vi "WPI_CANJaguar_SetMotor.vi"(8 "error in (no error)":errorcluster, 9 "options":u8, 10 "Output":dbl, 11 "MotorControlDevRef":T1={"DeviceStatus"={"status"=FALSE, "code"=0, "source"=""}, "Type"=enum."PWM", "PWM"={"PWM Channel"=enum."Invalid", "DeadBand"={"Name"="", "maxPositivePwm"=0, "minPositivePwm"=0, "centerPwm"=0, "maxNegativePwm"=0, "minNegativePwm"=0, "angularRange"=0}}, "CAN"={"Device Number"=0, "SetOutput VI Ref"=variant(refnum<vi> refnum), "GetOutput VI Ref"=variant(refnum<vi> refnum), "Enable VI Ref"=variant(refnum<vi> refnum), "Disable VI Ref"=variant(refnum<vi> refnum), "Data"=variant}, "Invert"=FALSE}) -> (0 "error out":errorcluster, 2 "Motor Output":dbl, 3 "MotorControlDevRef":T1={"DeviceStatus"={"status"=FALSE, "code"=0, "source"=""}, "Type"=enum."PWM", "PWM"={"PWM Channel"=enum."Invalid", "DeadBand"={"Name"="", "maxPositivePwm"=0, "minPositivePwm"=0, "centerPwm"=0, "maxNegativePwm"=0, "minNegativePwm"=0, "angularRange"=0}}, "CAN"={"Device Number"=0, "SetOutput VI Ref"=variant(refnum<vi> refnum), "GetOutput VI Ref"=variant(refnum<vi> refnum), "Enable VI Ref"=variant(refnum<vi> refnum), "Disable VI Ref"=variant(refnum<vi> refnum), "Data"=variant}, "Invert"=FALSE})   [LabVIEW 2016]
doc: "Specifies the output value or set-point for the motor controller.\n\nIf you use a motor controller connected to PWM, the scaled value can range from -1.0 to 1.0.\n\nIf you use a CAN Jaguar, the scale and the units depend on the mode the Jaguar is in. In <B>Percent VBus</B> mode, the range is the same as the PWM interface. In <B>Voltage</B>, <B>Current</B>, <B>Speed</B>, and <B>Position</B> modes, the <B>Output</B> is specified in engineering units (Volts, Amps, Rotations/Minute, and Rotations respectively).\n\nIf you use a CAN Talon SRX, the scale and the units depend on the mode the Talon SRXis in. In <B>Percent VBus</B> mode, the range is the same as the PWM interface. In <B>Speed</B>, and <B>Position</B> modes, the <B>Output</B> is specified in raw sensor units (ticks and ticks / 100 ms respectively).\n\nThis software is licensed. Open the labview\\readme\\WPI Robotics Library Open Source License.txt file for more information."
uses:
  <vilib>/Rock Robotics/WPI/MotorControl/WPI_MotorControlDeviceRef.ctl
  <vilib>/Rock Robotics/WPI/MotorControl/WPI_MotorControlType.ctl
  <vilib>/Rock Robotics/SystemInterfaces/DIO/FPGA_DIOPWMChannel.ctl
  <vilib>/Rock Robotics/WPI/PWM/WPI_PWMDeadband.ctl
  <vilib>/Rock Robotics/WPI/ThirdParty/CanMotor/CAN Jaguar/SubVIs/WPI_CANJaguar_RefNumData.ctl
  <vilib>/Rock Robotics/WPI/ThirdParty/CanMotor/CAN Jaguar/SubVIs/WPI_CANJaguar_ControlMode.ctl
  <vilib>/Rock Robotics/WPI/ThirdParty/CanMotor/CAN Jaguar/SubVIs/WPI_CAN_TokenMessageIDs.ctl
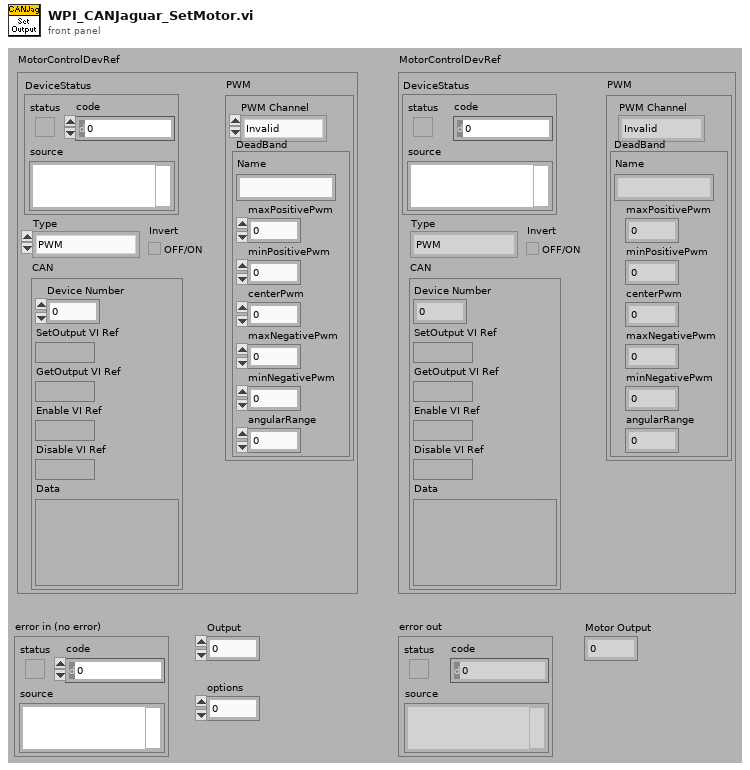
[diagram p1: front panel]
types:
  T1 = typedef "WPI_MotorControlDeviceRef.ctl" = cluster{"DeviceStatus":errorcluster, "Type":T2, "PWM":cluster{"PWM Channel":T3, "DeadBand":T4}, "CAN":cluster{"Device Number":u8, "SetOutput VI Ref":variant, "GetOutput VI Ref":variant, "Enable VI Ref":variant, "Disable VI Ref":variant, "Data":variant}, "Invert":bool}
  T2 = typedef "WPI_MotorControlType.ctl" = enum16{"PWM", "CAN"}
  T3 = typedef "FPGA_DIOPWMChannel.ctl" = enum8{"PWM 0", "PWM 1", "PWM 2", "PWM 3", "PWM 4", "PWM 5", "PWM 6", "PWM 7", "PWM 8", "PWM 9", "PWM MXP 0", "PWM MXP 1", "PWM MXP 2", "PWM MXP 3", "PWM MXP 4", "PWM MXP 5", "PWM MXP 6", "PWM MXP 7", "PWM MXP 8", "PWM MXP 9", "Invalid"}
  T4 = typedef "WPI_PWMDeadband.ctl" = cluster{"Name":string, "maxPositivePwm":i32, "minPositivePwm":i32, "centerPwm":i32, "maxNegativePwm":i32, "minNegativePwm":i32, "angularRange":u16}
  T5 = typedef "WPI_CANJaguar_RefNumData.ctl" = cluster{"CAN.Max Vout":dbl, "Control Mode":T6, "semaphore":T7}
  T6 = typedef "WPI_CANJaguar_ControlMode.ctl" = enum8{"Percent VBus", "Current", "Speed", "Position", "Voltage"}
  T7 = typedef "Semaphore RefNum" = refnum<k1>
  T8 = enum16{"big-endian, network order", "native, host order", "little-endian"}
  T9 = typedef "WPI_CAN_TokenMessageIDs.ctl" = u32
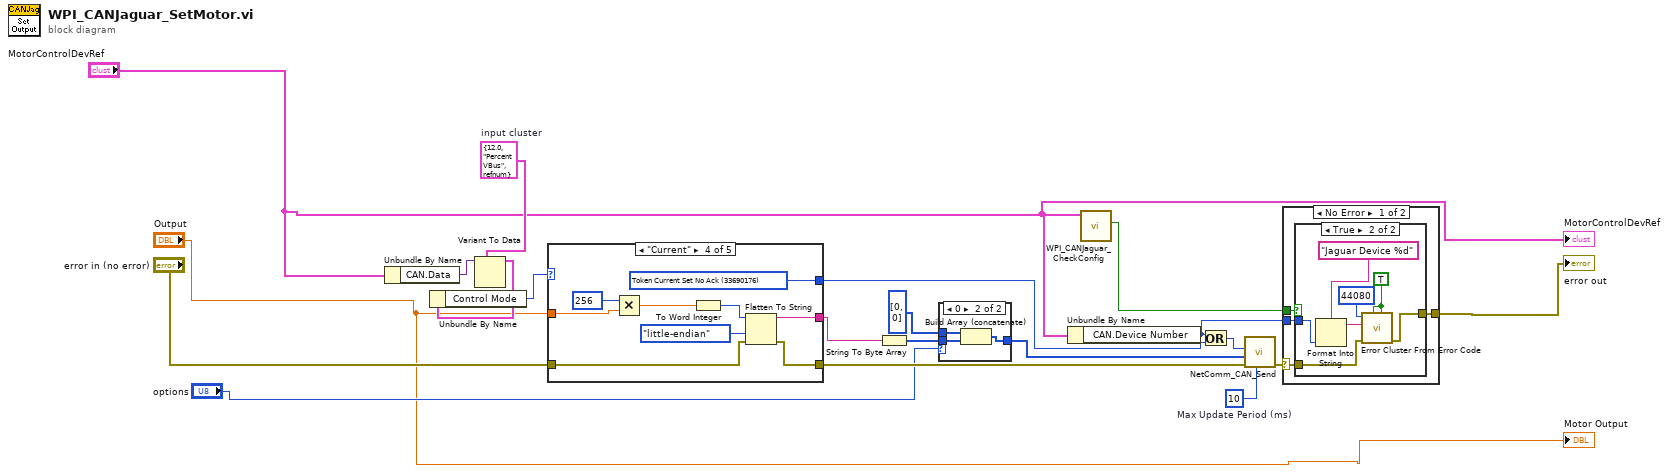
[diagram p0: block diagram]
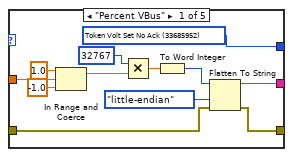
[diagram p4: hidden frame]
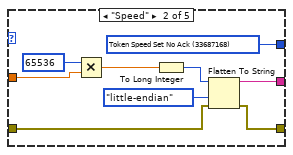
[diagram p5: hidden frame]
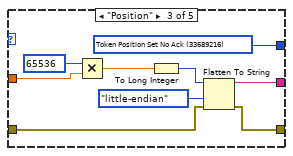
[diagram p6: hidden frame]
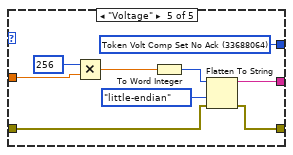
[diagram p7: hidden frame]
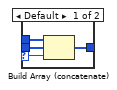
[diagram p8: hidden frame]
diagram:
  w8 = T5 {"CAN.Max Vout"=12.0, "Control Mode"=enum."Percent VBus", "semaphore"=refnum}  # input cluster
  w17 = 10  # Max Update Period (ms)
  n1 = Unbundle By Name("MotorControlDevRef") -> ("CAN.Data"=w9:variant)
  n2 = Variant To Data(type=w8, Variant=w9) -> (data=w7:T5)  [unwired: 1 in, 1 out]
  n3 = Unbundle By Name(w7) -> ("Control Mode"=w6:T6)
  n4 = case shown="\"Current\"" w6 {
    tunnel: [w21 w33 w42 w51 w60] -> w10
    tunnel: "Output" -> [w22 w35 w44 w54 w63]
    tunnel: "error in (no error)" -> [w29 w39 w47 w58 w67]
    tunnel: [w28 w38 w46 w57 w66] -> w12
    tunnel: [w23 w37 w48 w56 w65] -> w15
    frame "Percent VBus" {
      w21 = T9 33685952 items=["Token Volt Enable"=33685760, "Token Volt Set"=33685824, "Token Volt Set No Ack"=33685952, "Token Speed Enable"=33686976, "Token Speed Set"=33687040, "Token Speed Set No Ack"=33687168, "Token Volt Comp Enable"=33687872, "Token Volt Comp Set"=33687936, "Token Volt Comp Set No Ack"=33688064, "Token Position Enable"=33689024, "Token Position Set"=33689088, "Token Position Set No Ack"=33689216, "Token Current Enable"=33689984, "Token Current Set"=33690048, "Token Current Set No Ack"=33690176] ("CAN Token Message IDs")
      n5 = In Range and Coerce(upper limit=1.0, x=w22, lower limit=-1.0) -> (coerced(x)=w27:dbl)  [unwired: 1 out]
      n6 = Multiply(x=i16 32767, y=w27) -> (x*y=w25:dbl)
      n7 = To Word Integer(number=w25) -> (16bit integer=w24:i16)
      n8 = Flatten To String(anything=w24, byte order (0:big-endian, network order)=T8."little-endian", error in (no error)=w29) -> (data string=w23:string, error out=w28:errorcluster)  [unwired: 2 out]
    }
    frame "Speed" {
      w33 = T9 33687168 items=["Token Volt Enable"=33685760, "Token Volt Set"=33685824, "Token Volt Set No Ack"=33685952, "Token Speed Enable"=33686976, "Token Speed Set"=33687040, "Token Speed Set No Ack"=33687168, "Token Volt Comp Enable"=33687872, "Token Volt Comp Set"=33687936, "Token Volt Comp Set No Ack"=33688064, "Token Position Enable"=33689024, "Token Position Set"=33689088, "Token Position Set No Ack"=33689216, "Token Current Enable"=33689984, "Token Current Set"=33690048, "Token Current Set No Ack"=33690176] ("CAN Token Message IDs")
      n9 = Multiply(x=u32 65536, y=w35) -> (x*y=w34:dbl)
      n10 = To Long Integer(number=w34) -> (32bit integer=w41:i32)
      n11 = Flatten To String(anything=w41, byte order (0:big-endian, network order)=T8."little-endian", error in (no error)=w39) -> (data string=w37:string, error out=w38:errorcluster)  [unwired: 2 out]
    }
    frame "Position" {
      w42 = T9 33689216 items=["Token Volt Enable"=33685760, "Token Volt Set"=33685824, "Token Volt Set No Ack"=33685952, "Token Speed Enable"=33686976, "Token Speed Set"=33687040, "Token Speed Set No Ack"=33687168, "Token Volt Comp Enable"=33687872, "Token Volt Comp Set"=33687936, "Token Volt Comp Set No Ack"=33688064, "Token Position Enable"=33689024, "Token Position Set"=33689088, "Token Position Set No Ack"=33689216, "Token Current Enable"=33689984, "Token Current Set"=33690048, "Token Current Set No Ack"=33690176] ("CAN Token Message IDs")
      n12 = Multiply(x=u32 65536, y=w44) -> (x*y=w43:dbl)
      n13 = To Long Integer(number=w43) -> (32bit integer=w49:i32)
      n14 = Flatten To String(anything=w49, byte order (0:big-endian, network order)=T8."little-endian", error in (no error)=w47) -> (data string=w48:string, error out=w46:errorcluster)  [unwired: 2 out]
    }
    frame "Current" {
      w51 = T9 33690176 items=["Token Volt Enable"=33685760, "Token Volt Set"=33685824, "Token Volt Set No Ack"=33685952, "Token Speed Enable"=33686976, "Token Speed Set"=33687040, "Token Speed Set No Ack"=33687168, "Token Volt Comp Enable"=33687872, "Token Volt Comp Set"=33687936, "Token Volt Comp Set No Ack"=33688064, "Token Position Enable"=33689024, "Token Position Set"=33689088, "Token Position Set No Ack"=33689216, "Token Current Enable"=33689984, "Token Current Set"=33690048, "Token Current Set No Ack"=33690176] ("CAN Token Message IDs")
      n15 = Multiply(x=u32 256, y=w54) -> (x*y=w53:dbl)
      n16 = To Word Integer(number=w53) -> (16bit integer=w55:i16)
      n17 = Flatten To String(anything=w55, byte order (0:big-endian, network order)=T8."little-endian", error in (no error)=w58) -> (data string=w56:string, error out=w57:errorcluster)  [unwired: 2 out]
    }
    frame "Voltage" {
      w60 = T9 33688064 items=["Token Volt Enable"=33685760, "Token Volt Set"=33685824, "Token Volt Set No Ack"=33685952, "Token Speed Enable"=33686976, "Token Speed Set"=33687040, "Token Speed Set No Ack"=33687168, "Token Volt Comp Enable"=33687872, "Token Volt Comp Set"=33687936, "Token Volt Comp Set No Ack"=33688064, "Token Position Enable"=33689024, "Token Position Set"=33689088, "Token Position Set No Ack"=33689216, "Token Current Enable"=33689984, "Token Current Set"=33690048, "Token Current Set No Ack"=33690176] ("CAN Token Message IDs")
      n18 = Multiply(x=u32 256, y=w63) -> (x*y=w62:dbl)
      n19 = To Word Integer(number=w62) -> (16bit integer=w64:i16)
      n20 = Flatten To String(anything=w64, byte order (0:big-endian, network order)=T8."little-endian", error in (no error)=w67) -> (data string=w65:string, error out=w66:errorcluster)  [unwired: 2 out]
    }
  }
  n21 = String To Byte Array(string=w15) -> (unsigned byte array=w14:u8[])
  n22 = case shown="0" "options" {
    selector: "options" -> [w69 _]
    tunnel: [w72 w75] -> w11
    tunnel: u8[] [0, 0] ("data") -> [w71 w74]
    tunnel: w14 -> [w70 w73]
    frame Default {
      n23 = Build Array (concatenate)(w71, w70, w69) -> (w72:u8[])
    }
    frame 0 {
      n24 = Build Array (concatenate)(w74, w73) -> (w75:u8[])
    }
  }
  n25 = Unbundle By Name("MotorControlDevRef") -> ("CAN.Device Number"=w20:u8)
  n26 = call <vilib>:"WPI_CANJaguar_CheckConfig.vi"("CAN Jaguar Ref"="MotorControlDevRef") -> ("Warning"=w19:bool)  [unwired: 10 in]
  n27 = Or(x=w20, y=w10) -> (x .or. y?=w16:T9)
  n28 = call <vilib>:"NetComm_CAN_Send.vi"("Period (ms)"=w17, "error in (no error)"=w12, "Data"=w11, "Message ID"=w16) -> ("error out"=w18:errorcluster)  [unwired: 7 out]
  n29 = case shown="No Error" w18 {
    selector: w18 -> [w79 w88]
    tunnel: w19 -> [w76 _]
    tunnel: [w78 w88] -> w3
    tunnel: w20 -> [w77 _]
    frame No Error {
      n30 = case shown="True" w76 {
        tunnel: w79 -> [w80 w85]
        tunnel: [w80 w84] -> w78
        tunnel: w77 -> [_ w81]
        frame False {
        }
        frame True {
          w86 = TRUE ("is warning? (False)")
          n31 = Format Into String(format string="Jaguar Device %d", w81) -> (resulting string=w83:string)  [unwired: 2 in, 1 out]
          n32 = call <vilib>:"Error Cluster From Error Code.vi"("is warning? (False)"=w86, "show call chain? (False)"=w86, "error in (no error)"=w85, "error message (\"\")"=w83, "error code (0)"=44080) -> ("error out"=w84:errorcluster)  [unwired: 4 in]
        }
      }
    }
    frame Error {
    }
  }
  "error out" <- w3
  "MotorControlDevRef" <- "MotorControlDevRef"
  "Motor Output" <- "Output"
